vi "设置窗口.vi"() -> ()   [LabVIEW 2016]
uses:
  Holding Var.vi
panel:
  in  "多参数":T1={"水温"={"参数输入"={"采样模式"=enum."自动采样", "采样点数"=3, "变异系数设定值"=0.1, "重新取值百分比"=0.5, "偏差模式"=enum."相对偏差", "相对偏差百分比"=0.5, "绝对偏差值"=0.0}, "采样值"=[], "启用"=FALSE}, "pH"={"参数输入"={"采样模式"=enum."自动采样", "采样点数"=3, "变异系数设定值"=0.1, "重新取值百分比"=0.5, "偏差模式"=enum."相对偏差", "相对偏差百分比"=0.5, "绝对偏差值"=0.0}, "采样值"=[], "启用"=FALSE}, "DO%"={"参数输入"={"采样模式"=enum."自动采样", "采样点数"=3, "变异系数设定值"=0.1, "重新取值百分比"=0.5, "偏差模式"=enum."相对偏差", "相对偏差百分比"=0.5, "绝对偏差值"=0.0}, "采样值"=[], "启用"=FALSE}, "电导率"={"参数输入"={"采样模式"=enum."自动采样", "采样点数"=3, "变异系数设定值"=0.1, "重新取值百分比"=0.5, "偏差模式"=enum."相对偏差", "相对偏差百分比"=0.5, "绝对偏差值"=0.0}, "采样值"=[], "启用"=FALSE}, "浊度"={"参数输入"={"采样模式"=enum."自动采样", "采样点数"=3, "变异系数设定值"=0.1, "重新取值百分比"=0.5, "偏差模式"=enum."相对偏差", "相对偏差百分比"=0.5, "绝对偏差值"=0.0}, "采样值"=[], "启用"=FALSE}} {"浊度"."参数输入"."相对偏差百分比" format="%.2f%%"; "电导率"."参数输入"."相对偏差百分比" format="%.2f%%"; "DO%"."采样值" format="%.2f%%"; "DO%"."参数输入"."绝对偏差值" format="%.2f%%"; "DO%"."参数输入"."相对偏差百分比" format="%.2f%%"; "pH"."参数输入"."相对偏差百分比" format="%.2f%%"; "水温"."参数输入"."相对偏差百分比" format="%.2f%%"}
  in  "布尔":bool
  in  "控制模式":enum16{"手动", "自动"}(ring)
  in  "关闭时间（H）":u16
  in  "开启时间（H）":u16
  in  "总开关":bool
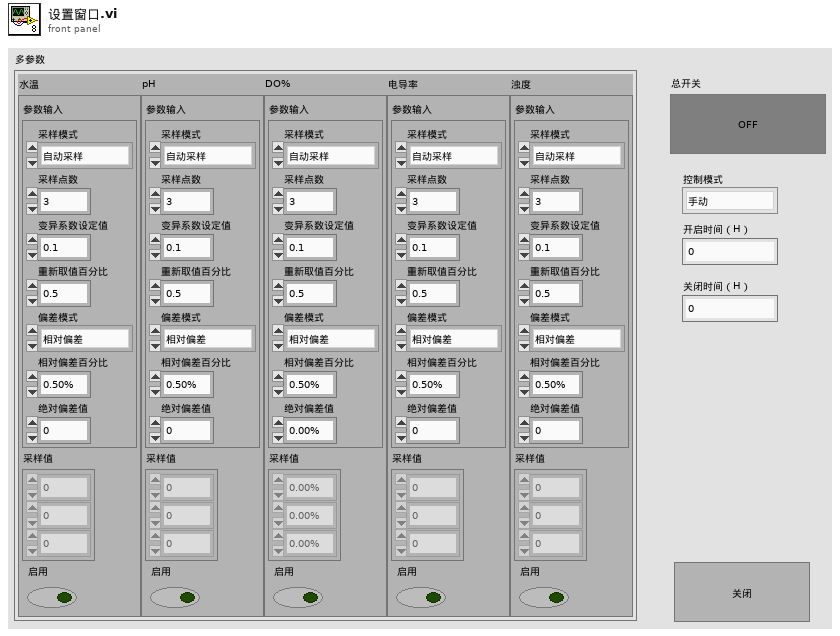
[diagram p1: front panel]
types:
  T1 = cluster{"水温":cluster{"参数输入":cluster{"采样模式":enum16{"自动采样", "手动采样"}, "采样点数":i32, "变异系数设定值":dbl, "重新取值百分比":dbl, "偏差模式":enum16{"相对偏差", "绝对偏差"}, "相对偏差百分比":dbl, "绝对偏差值":dbl}, "采样值":dbl[], "启用":bool}, "pH":cluster{"参数输入":cluster{"采样模式":enum16{"自动采样", "手动采样"}, "采样点数":i32, "变异系数设定值":dbl, "重新取值百分比":dbl, "偏差模式":enum16{"相对偏差", "绝对偏差"}, "相对偏差百分比":dbl, "绝对偏差值":dbl}, "采样值":dbl[], "启用":bool}, "DO%":cluster{"参数输入":cluster{"采样模式":enum16{"自动采样", "手动采样"}, "采样点数":i32, "变异系数设定值":dbl, "重新取值百分比":dbl, "偏差模式":enum16{"相对偏差", "绝对偏差"}, "相对偏差百分比":dbl, "绝对偏差值":dbl}, "采样值":dbl[], "启用":bool}, "电导率":cluster{"参数输入":cluster{"采样模式":enum16{"自动采样", "手动采样"}, "采样点数":i32, "变异系数设定值":dbl, "重新取值百分比":dbl, "偏差模式":enum16{"相对偏差", "绝对偏差"}, "相对偏差百分比":dbl, "绝对偏差值":dbl}, "采样值":dbl[], "启用":bool}, "浊度":cluster{"参数输入":cluster{"采样模式":enum16{"自动采样", "手动采样"}, "采样点数":i32, "变异系数设定值":dbl, "重新取值百分比":dbl, "偏差模式":enum16{"相对偏差", "绝对偏差"}, "相对偏差百分比":dbl, "绝对偏差值":dbl}, "采样值":dbl[], "启用":bool}}
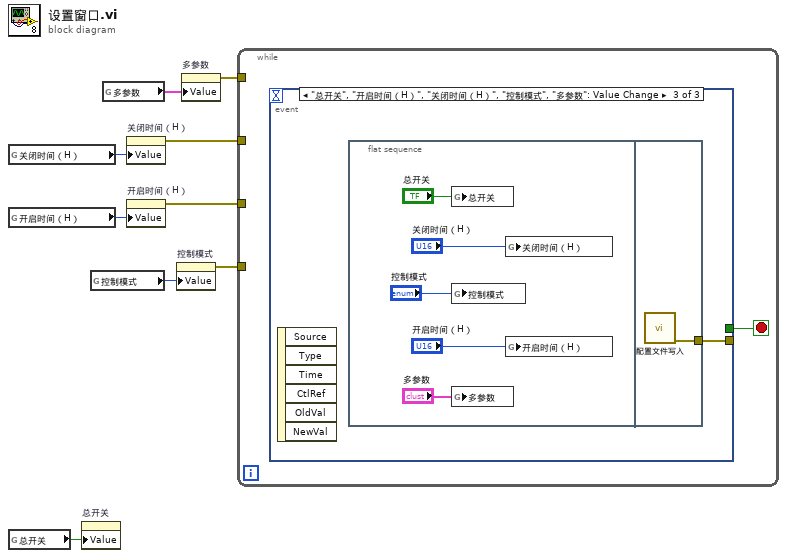
[diagram p0: block diagram]
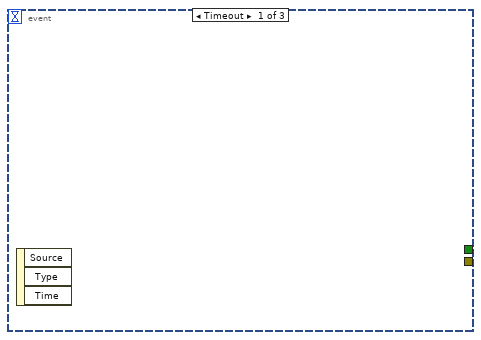
[diagram p2: hidden frame]
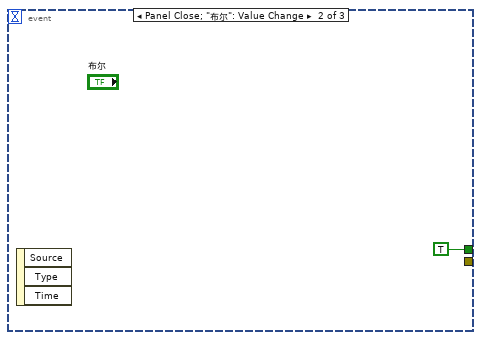
[diagram p3: hidden frame]
diagram:
  n1 = global read "Holding Var.vi" "关闭时间（H）"() -> (w6:u16)
  n2 = global read "Holding Var.vi" "开启时间（H）"() -> (w7:u16)
  n3 = global read "Holding Var.vi" "总开关"() -> (w9:bool)
  n4 = property on="总开关" class="Bool (strict)"("Value"=w9) -> ()  [unwired: 2 in, 2 out]
  n5 = global read "Holding Var.vi" "控制模式"() -> (w8:enum16{"手动", "自动"})
  n6 = global read "Holding Var.vi" "多参数"() -> (w2:T1)
  n7 = property on="关闭时间（H）" class="DigNum (strict)"("Value"=w6) -> (error out=w3:errorcluster)  [unwired: 2 in, 1 out]
  n8 = property on="开启时间（H）" class="DigNum (strict)"("Value"=w7) -> (error out=w4:errorcluster)  [unwired: 2 in, 1 out]
  n9 = property on="控制模式" class="Enum (strict)"("Value"=w8) -> (error out=w5:errorcluster)  [unwired: 2 in, 1 out]
  n10 = property on="多参数" class="Clust (strict)"("Value"=w2) -> (error out=w1:errorcluster)  [unwired: 2 in, 1 out]
  n11 = while {
    tunnel: w5 -> [_]
    tunnel: w4 -> [_]
    tunnel: w3 -> [_]
    tunnel: w1 -> [_]
    stop <- w10 stop-if-true
    n12 = event shown="[2] \"总开关\", \"开启时间（H）\", \"关闭时间（H）\", \"控制模式\", \"多参数\": Value Change" {
      selector: _ -> [_ _ _]
      dyn-events: _ -> [_ _ _]
      timeout: _ -> [_ _ _]
      tunnel: [_ TRUE _] -> w10
      tunnel: [_ _ w12] -> _
      event Timeout {
        n13 = event-data() -> ()  [unwired: 1 in, 3 out]
      }
      event Panel Close; "布尔": Value Change {
        n14 = event-data() -> ()  [unwired: 1 in, 3 out]
      }
      event "总开关", "开启时间（H）", "关闭时间（H）", "控制模式", "多参数": Value Change {
        n15 = event-data() -> ()  [unwired: 1 in, 6 out]
        n16 = flat-sequence {
          tunnel: [w18] -> w12
          frame #0 {
            n17 = global write "Holding Var.vi" "总开关"("总开关") -> ()
            n18 = global write "Holding Var.vi" "控制模式"("控制模式") -> ()
            n19 = global write "Holding Var.vi" "多参数"("多参数") -> ()
            n20 = global write "Holding Var.vi" "关闭时间（H）"("关闭时间（H）") -> ()
            n21 = global write "Holding Var.vi" "开启时间（H）"("开启时间（H）") -> ()
          }
          frame #1 {
            n22 = call "配置文件写入.vi"() -> ("错误输出"=w18:errorcluster)  [unwired: 11 in]
          }
        }
      }
    }
  }
